vi "Harmonics MSMT Configure DPD.vi"(8 "error in (no error)":errorcluster, 10 "Step In":refnum<k7>, 11 "Harmonics in":refnum<class "Harmonics.lvclass">) -> (0 "error out":errorcluster, 2 "Step Out":refnum<k7>, 3 "Harmonics out":refnum<class "Harmonics.lvclass">)   [LabVIEW 2018, in "Harmonics.lvlib" / "Harmonics.lvclass"]
uses:
  Harmonics.lvclass
  Plugins/String Database.lvlibp/String Database.lvclass
  Plugins/Test Group Manager.lvlibp/Test Group Manager.lvclass
  Plugins/Test Group Manager.lvlibp/Includes/Test Group/Test Group.lvclass
  Plugins/TestStand API Tools (TSAT).lvlibp/Step Actions/TSAT Step Actions.lvlib
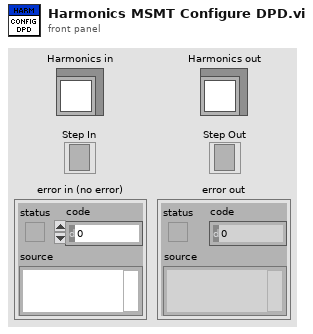
[diagram p1: front panel]
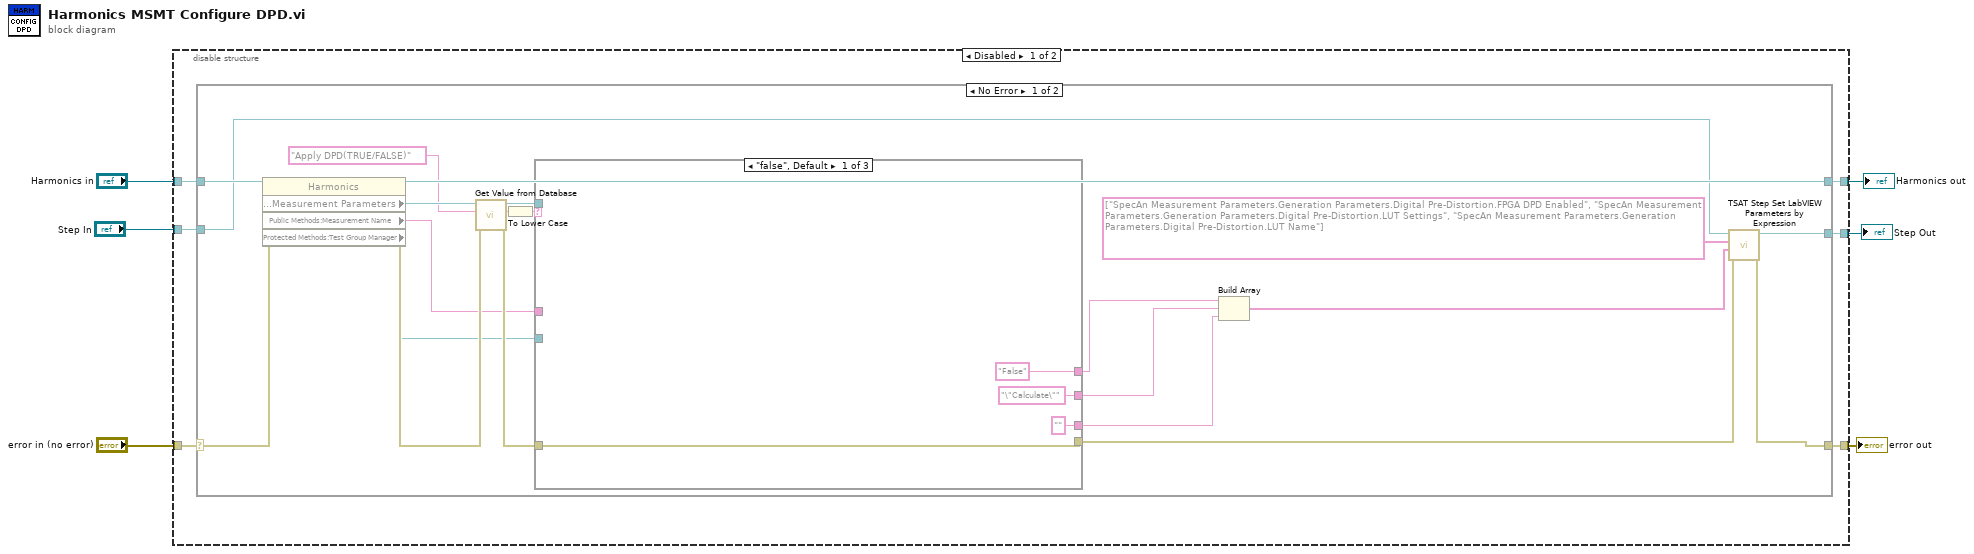
[diagram p0: block diagram]
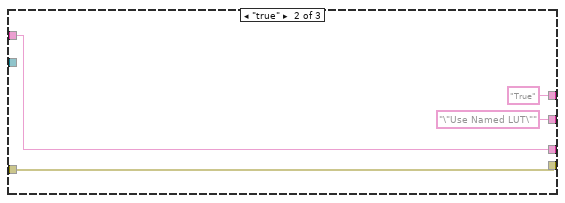
[diagram p2: hidden frame]
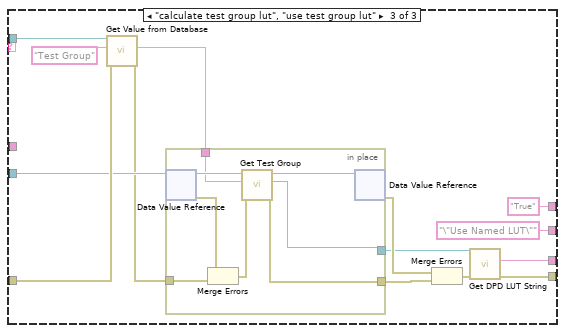
[diagram p3: hidden frame]
diagram:
  n1 = disable-structure shown="Disabled" {
    disable-tunnel: "error in (no error)" -> [w12 _]
    disable-tunnel: [w11 _] -> w5
    disable-tunnel: "Harmonics in" -> [w10 _]
    disable-tunnel: [w9 _] -> w3
    disable-tunnel: [w8 _] -> w2
    disable-tunnel: "Step In" -> [w7 _]
    frame Disabled {
      n2 = case shown="No Error" w12 {
        selector: w12 -> [w33 w66]
        tunnel: [w23 w66] -> w11
        tunnel: [w31 w65] -> w9
        tunnel: w10 -> [w32 w65]
        tunnel: [w15 w64] -> w8
        tunnel: w7 -> [w14 w64]
        frame No Error {
          n3 = property class="Harmonics"(reference=w32, error in=w33) -> (reference out=w31:refnum<class "Harmonics.lvclass">, error out=w29:errorcluster, "Protected Methods:Measurement Parameters"=w30:refnum<class "String Database.lvclass">, "Public Methods:Measurement Name"=w16:string, "Protected Methods:Test Group Manager"=w24:refnum<data-value>)
          n4 = call "Get Value from Database.vi"("error in (no error)"=w29, "Entry Name"="Apply DPD(TRUE/FALSE)", "Message in"=w30) -> ("error out"=w26:errorcluster, "Entry Value"=w27:string, "Message out"=w25:refnum<class "String Database.lvclass">)  [unwired: 5 in, 1 out]
          n5 = To Lower Case(string=w27) -> (all lower case string=w13:string)
          n6 = case shown="\"false\", Default" w13 {
            tunnel: w26 -> [w37 w41 w54]
            tunnel: w25 -> [_ _ w55]
            tunnel: w24 -> [_ _ w52]
            tunnel: ["" ("DPD LUT") w38 w45] -> w19
            tunnel: [w37 w41 w44] -> w22
            tunnel: ["False" "True" "True"] -> w21
            tunnel: ["\"Calculate\"" "\"Use Named LUT\"" "\"Use Named LUT\""] -> w20
            tunnel: w16 -> [_ w38 _]
            frame "false", Default {
            }
            frame "true" {
            }
            frame "calculate test group lut", "use test group lut" {
              n7 = call "Get Value from Database.vi"("error in (no error)"=w54, "Entry Name"="Test Group", "Message in"=w55) -> ("error out"=w51:errorcluster, "Entry Value"=w50:string)  [unwired: 5 in, 2 out]
              n8 = in-place {
                in-place-border: w51 -> [w60]
                in-place-border: w50 -> [w62]
                in-place-border: [w57] -> w48
                in-place-border: [w56] -> w46
                n9 = in-place-dvr #1(w52) -> (w63:refnum<class "Test Group Manager.lvclass">, w58:errorcluster)
                n10 = Merge Errors(w58, w60) -> (w59:errorcluster)
                n11 = call "Get Test Group.vi"("error in (no error)"=w59, "Test Group Name"=w62, "Test Group Manager in"=w63) -> ("error out"=w57:errorcluster, "Test Group In"=w56:refnum<data-value>, "Test Group Manager out"=w61:refnum<class "Test Group Manager.lvclass">)  [unwired: 6 in]
                n12 = in-place-dvr #1(w61) -> (w49:errorcluster)  [unwired: 1 out]
              }
              n13 = Merge Errors(w49, w48) -> (w47:errorcluster)
              n14 = call "Get DPD LUT String.vi"("error in (no error)"=w47, "Test Group In"=w46) -> ("error out"=w44:errorcluster, "DPD LUT"=w45:string)  [unwired: 7 in, 1 out]
            }
          }
          n15 = Build Array(w21, w20, w19) -> (w18:string[])
          n16 = call "TSAT Step Set LabVIEW Parameters by Expression.vi"("Error In"=w22, "Value Expressions"=w18, "Parameters to Set"=string[] ["SpecAn Measurement Parameters.Generation Parameters.Digital Pre-Distortion.FPGA DPD Enabled", "SpecAn Measurement Parameters.Generation Parameters.Digital Pre-Distortion.LUT Settings", "SpecAn Measurement Parameters.Generation Parameters.Digital Pre-Distortion.LUT Name"], "Step In"=w14) -> ("Error Out"=w23:errorcluster, "Step Out"=w15:refnum<k7>)  [unwired: 6 in]
        }
        frame Error {
        }
      }
    }
    frame Enabled {
    }
  }
  "error out" <- w5
  "Harmonics out" <- w3
  "Step Out" <- w2
